vi "dfd_Error Cluster From Error Code (Scalar).vi"(8 "error in (no error)":errorcluster, 11 "error code (0)":i32) -> (0 "error out":errorcluster)   [LabVIEW 2017, in "NI_DigFilterLicensed.lvlib"]
uses:
  <vilib>/addons/Digital Filter Design/NI_DigFilterLicensed.lvlib
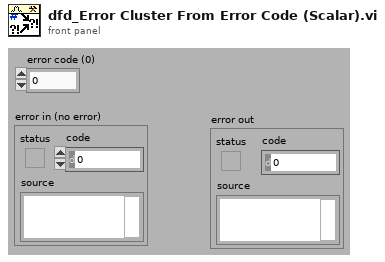
[diagram p1: front panel]
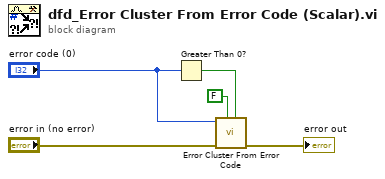
[diagram p0: block diagram]
diagram:
  n1 = Greater Than 0?(x="error code (0)") -> (x > 0?=w5:bool)
  n2 = call <vilib>:"Error Cluster From Error Code.vi"("is warning? (False)"=w5, "show call chain? (False)"=FALSE, "error in (no error)"="error in (no error)", "error code (0)"="error code (0)") -> ("error out"=→"error out":errorcluster)  [unwired: 5 out]
